vi "TestLoad.vi"() -> ()   [LabVIEW 2019]
uses:
  TestSeqClass.lvclass
  GUIHandler/GUI_Handler.lvclass
panel:
  in  "GUI_Handler.lvclass":refnum<class "GUI_Handler.lvclass">
  in  "TestSeqClass.lvclass":refnum<class "TestSeqClass.lvclass">
  in  "Multicolumn Listbox":i32(listbox)
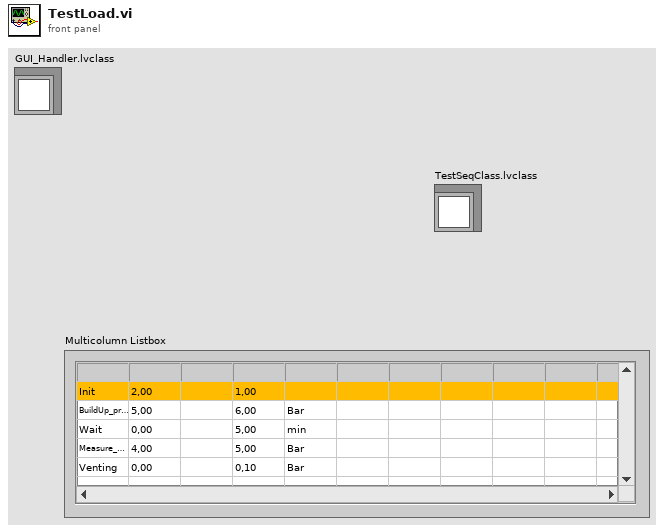
[diagram p1: front panel]
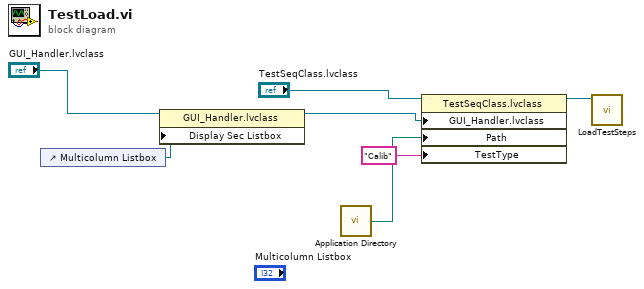
[diagram p0: block diagram]
diagram:
  n1 = control-ref of="Multicolumn Listbox"() -> (w2:refnum<vi>)
  n2 = property class="GUI_Handler.lvclass"(reference="GUI_Handler.lvclass", "Display Sec Listbox"=w2) -> (reference out=w1:refnum<class "GUI_Handler.lvclass">)  [unwired: 1 in, 1 out]
  n3 = call <vilib>:"Application Directory.vi"() -> ("Application Directory"=w5:path)
  n4 = property class="TestSeqClass.lvclass"(reference="TestSeqClass.lvclass", "GUI_Handler.lvclass"=w1, "Path"=w5, "TestType"="Calib") -> (reference out=w7:refnum<class "TestSeqClass.lvclass">)  [unwired: 1 in, 1 out]
  n5 = call-dynamic "LoadTestSteps.vi"("TestSeqClass in"=w7) -> ()  [unwired: 9 in, 2 out]
